vi "BPSK_ber.vi"(8 "error in":errorcluster, 9 "rxbit":cdb[](array[numeric]), 10 "txbit":cdb[](array[numeric]), 11 "Path In":path) -> (0 "error out":errorcluster, 1 "ber":dbl, 2 "errnum":dbl, 3 "Path Out":path)   [LabVIEW 2015]
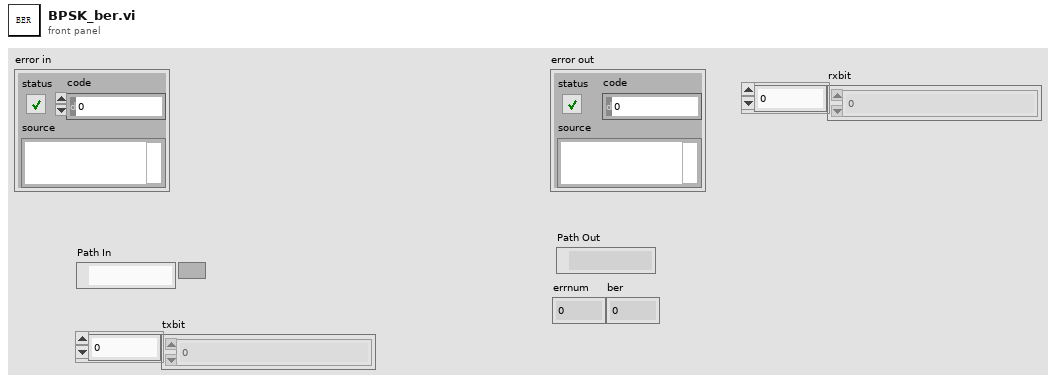
[diagram p1: front panel]
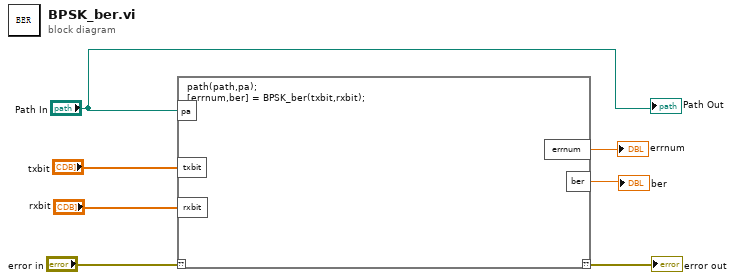
[diagram p0: block diagram]
diagram:
  n1 = script code="path(path,pa);\n[errnum,ber] = BPSK_ber(txbit,rxbit);"("??"="error in", "pa"="Path In", "txbit"="txbit", "rxbit"="rxbit") -> ("??"=→"error out":errorcluster, "errnum"=→"errnum":dbl, "ber"=→"ber":dbl)
  "Path Out" <- "Path In"
